vi "loadTriggeringInUse.vi"(6 "type":string, 8 "error in (no error)":errorcluster, 9 "device.lvclass":refnum<class "device.lvclass">, 10 "NativeXML in":refnum<class "NativeXML.lvclass">, 11 "deviceDataBase in":refnum<class "deviceDataBase.lvclass">) -> (0 "error out":errorcluster, 1 "device.lvclass out":refnum<class "device.lvclass">, 2 "NativeXML out":refnum<class "NativeXML.lvclass">, 3 "deviceDataBase out":refnum<class "deviceDataBase.lvclass">)   [LabVIEW 2011, in "Tools.lvlib" / "DatabaseHelpers.lvlib" / "deviceDataBase.lvclass"]
uses:
  deviceDataBase.lvclass
  NativeXML/NativeXML.lvclass
  Database Objects/device/device.lvclass
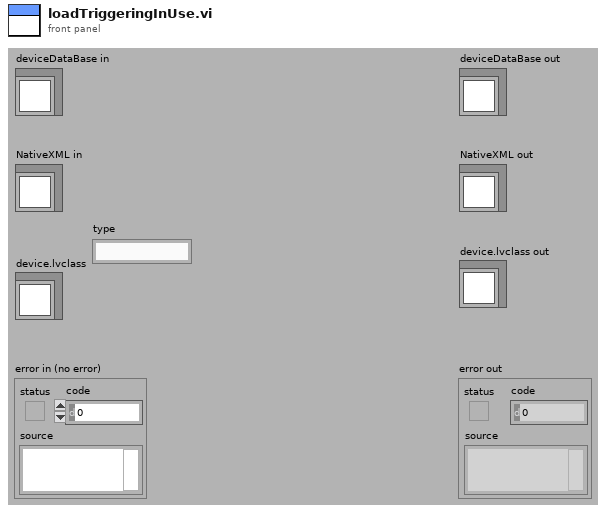
[diagram p1: front panel]
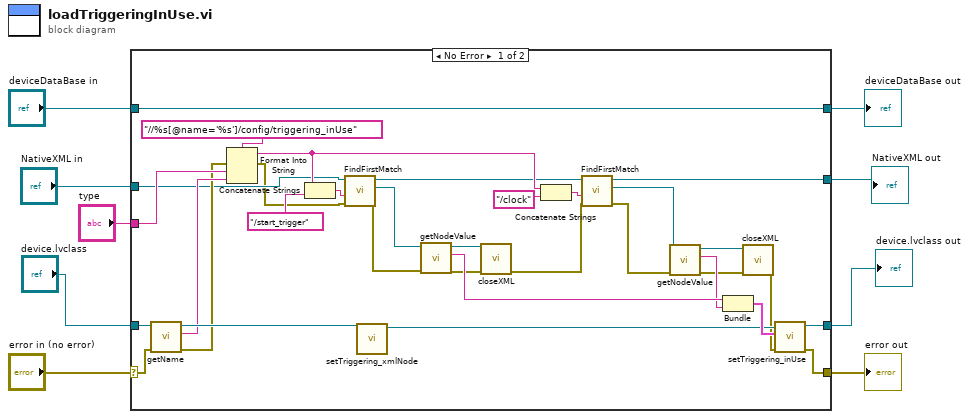
[diagram p0: block diagram]
diagram:
  n1 = case shown="No Error" "error in (no error)" {
    selector: "error in (no error)" -> [w33 w44]
    tunnel: [w40 w44] -> w8
    tunnel: [w42 w43] -> w6
    tunnel: "deviceDataBase in" -> [w42 w43]
    tunnel: "NativeXML in" -> [w17 _]
    tunnel: "device.lvclass" -> [w35 _]
    tunnel: [w39 _] -> w3
    tunnel: "type" -> [w32 _]
    tunnel: [w12 _] -> w1
    frame No Error {
      n2 = call "getName.vi"("error in (no error)"=w33, "device.lvclass in"=w35) -> ("error out"=w30:errorcluster, "name"=w31:string, "device.lvclass out"=w34:refnum<class "device.lvclass">)  [unwired: 7 in]
      n3 = Format Into String(format string="//%s[@name='%s']/config/triggering_inUse", error in=w30, w32, w31) -> (resulting string=w20:string, error out=w14:errorcluster)  [unwired: 1 in]
      n4 = Concatenate Strings(w20, "/start_trigger") -> (w24:string)
      n5 = call "FindFirstMatch.vi"("error in (no error)"=w14, "xPath"=w24, "NativeXML in"=w17) -> ("error out"=w15:errorcluster, "NativeXML match"=w16:refnum<class "NativeXML.lvclass">, "NativeXML out"=w18:refnum<class "NativeXML.lvclass">)  [unwired: 6 in]
      n6 = call "setTriggering_xmlNode.vi"("device.lvclass in"=w34) -> ("device.lvclass out"=w38:refnum<class "device.lvclass">)  [unwired: 9 in, 1 out]
      n7 = call "getNodeValue.vi"("error in (no error)"=w15, "NativeXML in"=w16) -> ("error out"=w29:errorcluster, "Value"=w37:string, "NativeXML out"=w28:refnum<class "NativeXML.lvclass">)  [unwired: 7 in]
      n8 = call "closeXML.vi"("error in (no error)"=w29, "NativeXML in"=w28) -> ("error out"=w13:errorcluster)  [unwired: 9 in]
      n9 = Concatenate Strings(w20, "/clock") -> (w21:string)
      n10 = call "FindFirstMatch.vi"("error in (no error)"=w13, "xPath"=w21, "NativeXML in"=w18) -> ("error out"=w10:errorcluster, "NativeXML match"=w11:refnum<class "NativeXML.lvclass">, "NativeXML out"=w12:refnum<class "NativeXML.lvclass">)  [unwired: 6 in]
      n11 = call "getNodeValue.vi"("error in (no error)"=w10, "NativeXML in"=w11) -> ("error out"=w27:errorcluster, "Value"=w36:string, "NativeXML out"=w26:refnum<class "NativeXML.lvclass">)  [unwired: 7 in]
      n12 = Bundle("Value"=w37, "Value"=w36) -> (w41:cluster{"Value":string, "Value":string})  [unwired: 1 in]
      n13 = call "closeXML.vi"("error in (no error)"=w27, "NativeXML in"=w26) -> ("error out"=w25:errorcluster)  [unwired: 9 in]
      n14 = call "setTriggering_inUse.vi"("error in (no error)"=w25, "triggering_inUse"=w41, "device.lvclass in"=w38) -> ("error out"=w40:errorcluster, "device.lvclass out"=w39:refnum<class "device.lvclass">)  [unwired: 7 in]
    }
    frame Error {
    }
  }
  "error out" <- w8
  "deviceDataBase out" <- w6
  "NativeXML out" <- w1
  "device.lvclass out" <- w3
